vi "Initialise folders.vi"(8 "error in (no error)":errorcluster) -> (0 "error out":errorcluster)   [LabVIEW 2017]
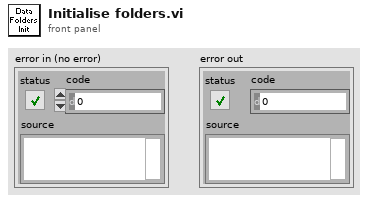
[diagram p1: front panel]
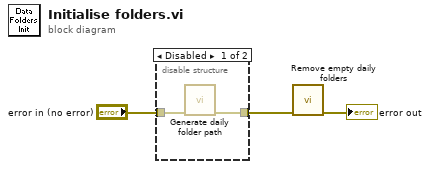
[diagram p0: block diagram]
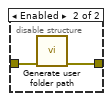
[diagram p2: hidden frame]
diagram:
  n1 = disable-structure shown="Disabled" {
    disable-tunnel: [w5 w6] -> w3
    disable-tunnel: "error in (no error)" -> [w4 w7]
    frame Disabled {
      n2 = call "Generate daily folder path.vi"("error in (no error)"=w4) -> ("error out"=w5:errorcluster)  [unwired: 10 in]
    }
    frame Enabled {
      n3 = call "Generate user folder path.vi"("error in (no error)"=w7) -> ("error out"=w6:errorcluster)  [unwired: 9 in, 1 out]
    }
  }
  n4 = call "Remove empty daily folders.vi"("error in (no error)"=w3) -> ("error out"=→"error out":errorcluster)  [unwired: 10 in]
